vi "receive_data.vi"(3 "error in":errorcluster, 4 "header size":i8, 5 "connection ID":refnum<k5>) -> (0 "error out":errorcluster, 1 "data out":string, 2 "connection ID out":refnum<k5>)   [LabVIEW 2018]
panel:
  out "number":i8
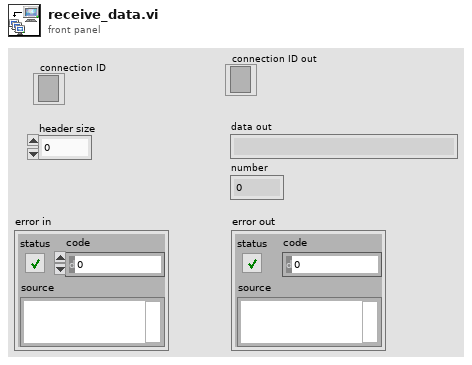
[diagram p1: front panel]
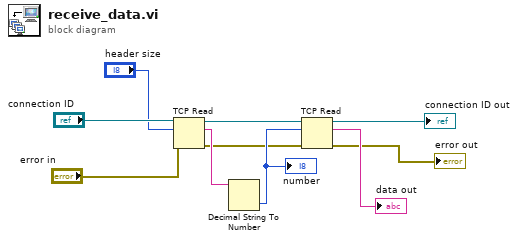
[diagram p0: block diagram]
diagram:
  n1 = TCP Read(connection ID="connection ID", bytes to read="header size", error in (no error)="error in") -> (connection ID out=w6:refnum<k5>, data out=w7:string, error out=w4:errorcluster)  [unwired: 2 in]
  n2 = Decimal String To Number(string=w7) -> (number=w5:i32)  [unwired: 2 in, 1 out]
  "number" <- w5
  n3 = TCP Read(connection ID=w6, bytes to read=w5, error in (no error)=w4) -> (connection ID out=→"connection ID out":refnum<k5>, data out=→"data out":string, error out=→"error out":errorcluster)  [unwired: 2 in]
